vi "Convert Analog PWM Values to Analog Measurement.vi"(9 "Length":i32, 10 "Index":i32, 11 "Channel Values in":dbl[](array[numeric])) -> (2 "Settings":T1, 3 "Channel Values out":dbl[](array[numeric]))   [LabVIEW 2018, in "FPGA Addon Engine.lvlib"]
uses:
  FPGA Addon Engine.lvlib
  Submodules/Source/Types/PWM.Measure.Analog.Settings.ctl
  Submodules/Source/Speciality FPGA IO.lvlib
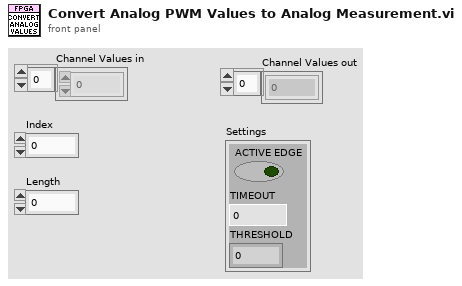
[diagram p1: front panel]
types:
  T1 = typedef "Speciality FPGA IO.lvlib/PWM.Measure.Analog.Settings.ctl" = cluster{"ACTIVE EDGE":bool, "TIMEOUT":u32, "THRESHOLD":fxp<+/-,32,8>}
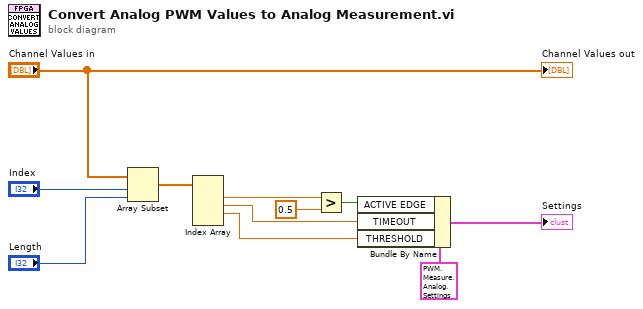
[diagram p0: block diagram]
diagram:
  n1 = Array Subset(array="Channel Values in", index="Index", length="Length") -> (w1:dbl[])
  n2 = Index Array(array=w1) -> (element #1=w3:dbl, element #2=w5:dbl, element #3=w6:dbl)  [unwired: 4 in, 1 out]
  n3 = Greater?(x=w3, y=0.5) -> (0:w4:bool)
  n4 = Bundle By Name(cluster=T1 {"ACTIVE EDGE"=FALSE, "TIMEOUT"=0, "THRESHOLD"=0.0}, "ACTIVE EDGE"=w4, "TIMEOUT"=w5, "THRESHOLD"=w6) -> (→"Settings":T1)
  "Channel Values out" <- "Channel Values in"
